vi "Close.vi"(8 "error in (no error)":errorcluster caption="错误输入（无错误）", 11 "ZLGCAN 输入":refnum<class "ZLGCAN.lvclass">) -> (0 "error out":errorcluster caption="错误输出", 3 "ZLGCAN 输出":refnum<class "ZLGCAN.lvclass">)   [LabVIEW 2020, in "ZLGCAN.lvclass"]
uses:
  ZLGCAN.lvclass
  ZLGCAN.lvclass/ZLGCAN.ctl
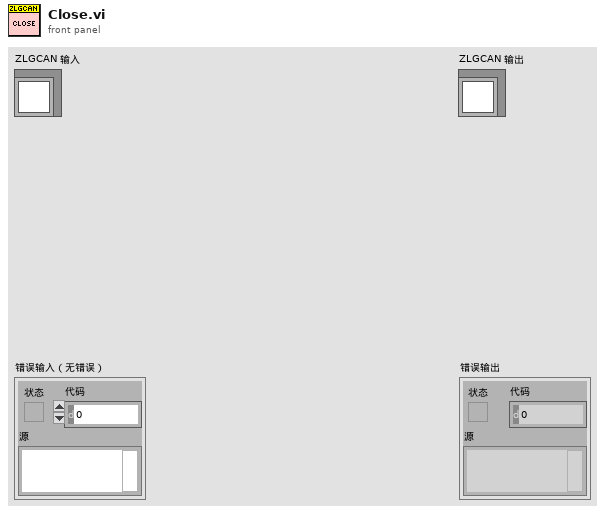
[diagram p1: front panel]
types:
  T1 = cluster{"Device Type":u32, "Device Index":u32, "CANInd":u32, "Baud(E_U)":u32}
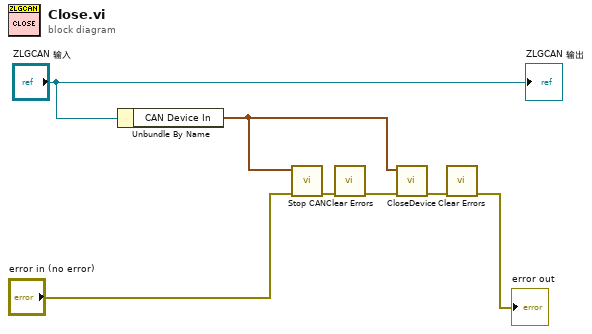
[diagram p0: block diagram]
diagram:
  n1 = Unbundle By Name("ZLGCAN 输入") -> ("CAN Device In"=w3:T1)
  n2 = call "Stop CAN.vi"("错误输入（无错误）"="error in (no error)", "CAN Device In"=w3) -> ("错误输出"=w7:errorcluster)  [unwired: 9 in]
  n3 = call <vilib>:"Clear Errors.vi"("error in (no error)"=w7) -> ("error out"=w2:errorcluster)  [unwired: 5 in, 1 out]
  n4 = call "CloseDevice.vi"("错误输入（无错误）"=w2, "CAN Device In"=w3) -> ("错误输出"=w4:errorcluster)  [unwired: 9 in]
  n5 = call <vilib>:"Clear Errors.vi"("error in (no error)"=w4) -> ("error out"=→"error out":errorcluster)  [unwired: 5 in, 1 out]
  "ZLGCAN 输出" <- "ZLGCAN 输入"
